vi "wav Crest Factor Analyzer.vi"() -> ()   [LabVIEW 2014]
doc: "This example demonstrates the effect of resampling a waveform in single-shot mode and the impact of the different resampling parameters. Single-shot mode is used when resampling a single block of the signal. Continuous mode is used when resampling separate but contiguous blocks of the signal."
uses:
  <vilib>/sound2/lvsound2.llb/Sound File Info (path).vi
  <vilib>/sound2/lvsound2.llb/Sound File Read Open.vi
  <vilib>/sound2/lvsound2.llb/Sound File Read (DBL).vi
  <vilib>/measure/maspectr.llb/FFT Spectrum (Mag-Phase) for N Chan.vi
  <vilib>/Utility/file.llb/Write To Spreadsheet File (string).vi
  <vilib>/Analysis/NI_AALPro.lvlib
  <vilib>/measure/NI_MAPro.lvlib
panel:
  in  "Auto Y":bool
  out "wav path":path
  out "FFT":cluster{"frequency":dbl[], "magnitude":dbl[]}[](graph)
  out "Result":string[][](array[string])
  in  "Tab Control":enum32{"General"}(tab)
  in  "Save":bool
  out "Progress bar":dbl(slide) scale=0.0..1.0
  in  "Analyze":bool
  out "Total no. of samples/ch":u32 format="%#_3p"
  out "Report path":path
  in  "Exit":bool
  in  "Smoothing":u16(ring)=3 items=["None"=0, "1/3 octave"=3, "1/6 octave"=6, "1/12 octave"=12, "1/24 octave"=24, "1/48 octave"=48]
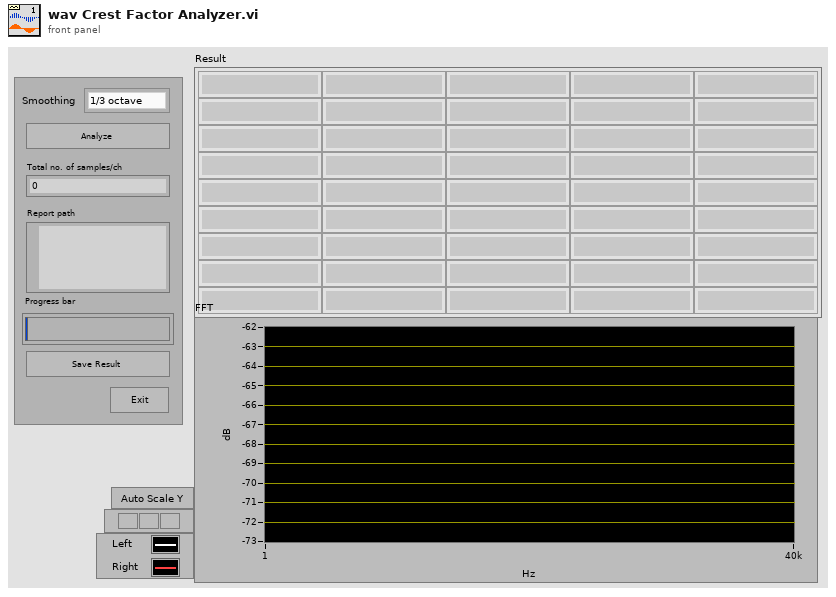
[diagram p1: front panel]
types:
  T1 = cluster{"averaging mode":enum16{"No averaging", "Vector averaging", "RMS averaging", "Peak hold"}, "weighting mode":enum16{"Linear", "Exponential"}, "number of averages":u32}
  T2 = cluster{"dB On (F)":bool, "unwrap phase (F)":bool, "convert to degree (F)":bool}
  T3 = typedef "Sound File Refnum.ctl" = refnum<file>
  T4 = typedef "imagedata.ctl" = cluster{"image type":i32, "image depth":i32, "image":u8[], "mask":u8[], "colors":u32[], "Rectangle":cluster{"left":i16, "top":i16, "right":i16, "bottom":i16}}
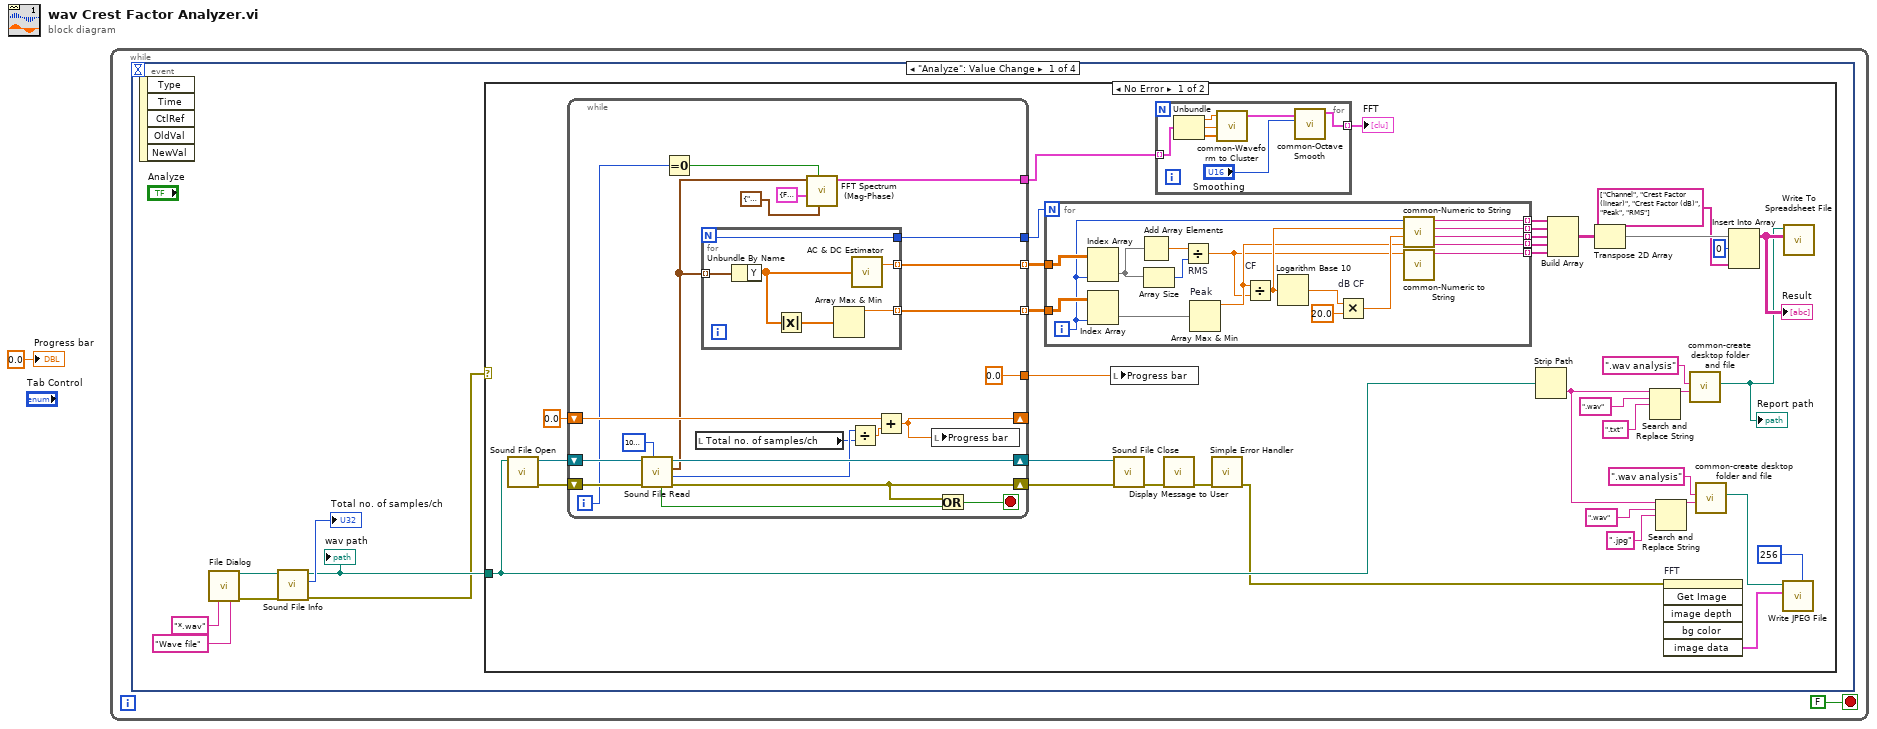
[diagram p0: block diagram]
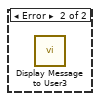
[diagram p2: hidden frame]
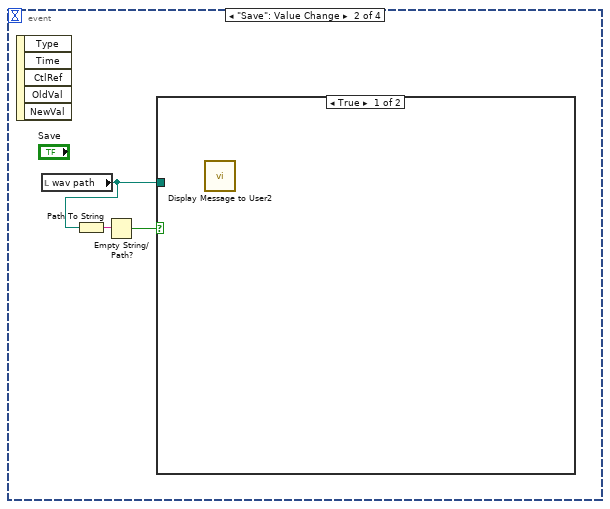
[diagram p3: hidden frame]
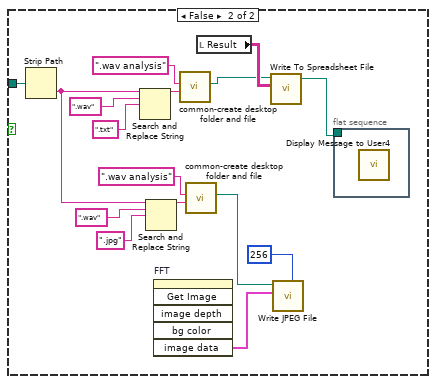
[diagram p4: hidden frame]
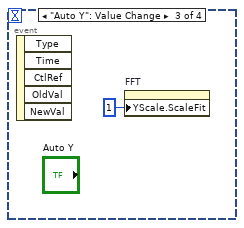
[diagram p5: hidden frame]
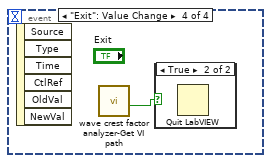
[diagram p6: hidden frame]
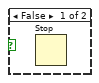
[diagram p7: hidden frame]
diagram:
  n1 = while {
    stop <- FALSE stop-if-true
    n2 = event shown="[0] \"Analyze\": Value Change" {
      selector: _ -> [_ _ _ _]
      dyn-events: _ -> [_ _ _ _]
      timeout: _ -> [_ _ _ _]
      event "Analyze": Value Change {
        n3 = event-data() -> ()  [unwired: 6 out]
        n4 = call "File Dialog"("pattern (all files)"="*.wav" ("pattern label"), "pattern label"="Wave file") -> ("selected path"=w7:path, "error out"=w4:errorcluster)  [unwired: 5 in, 7 out]
        n5 = call-poly <vilib>:"Sound File Info.vi"("error in (no error)"=w4, "path"=w7) -> ("error out"=w3:errorcluster, "total number of samples/ch"=→"Total no. of samples/ch":u32, "path out"=w5:path)  [unwired: 7 out]
        "wav path" <- w5
        n6 = case shown="No Error" w3 {
          tunnel: w5 -> [w22 _]
          frame No Error {
            n7 = call-poly <vilib>:"Sound File Open.vi"("path"=w22) -> ("error out"=w45:errorcluster, "sound file refnum"=w44:T3)  [unwired: 1 in, 8 out]
            n8 = while {
              shift-right: [w93] -> w47
              shift-left: w44 -> [w94]
              shift-right: [w75] -> w46
              shift-left: w45 -> [w92]
              shift-right: [w85] -> _
              shift-left: 0.0 ("Progress bar") -> [w90]
              tunnel: [0.0 ("Progress bar")] -> w42
              tunnel: [w84] -> w39 mode=indexing
              tunnel: [w83] -> w40 mode=indexing
              tunnel: [w82] -> w41
              tunnel: [w73] -> w10
              i -> [w80]
              stop <- w74 stop-if-true
              n9 = call-poly <vilib>:"Sound File Read.vi"("number of samples/ch (-1: all)"=1000000, "error in (no error)"=w92, "sound file refnum"=w94) -> ("error out"=w75:errorcluster, "offset"=w88:i32, "data"=w81:waveform(dbl)[], "sound file refnum out"=w93:T3, "end of file?"=w76:bool)  [unwired: 2 in, 2 out]
              n10 = Equal To 0?(x=w80) -> (x = 0?=w79:bool)
              n11 = local read "Total no. of samples/ch"() -> (w87:u32)
              n12 = for {
                N -> [w98]
                tunnel: w81 -> [w100] mode=indexing
                tunnel: [w99] -> w83 mode=indexing
                tunnel: [w97] -> w84 mode=indexing
                tunnel: [w98] -> w82
                n13 = Unbundle By Name(w100) -> ("Y"=w96:dbl[])
                n14 = Absolute Value(x=w96) -> (abs(x)=w95:dbl[])
                n15 = Array Max & Min(array=w95) -> (max value=w97:dbl)  [unwired: 3 out]
                n16 = call <vilib>:"AC & DC Estimator.vi"("Signal (V)"=w96) -> ("AC estimate (Vrms)"=w99:dbl)  [unwired: 1 out]
              }
              n17 = call-poly <vilib>:"FFT Spectrum (Mag-Phase).vi"("averaging parameters"=T1 {"averaging mode"=enum."No averaging", "weighting mode"=enum."Linear", "number of averages"=99999}, "restart averaging (F)"=w79, "view"=T2 {"dB On (F)"=FALSE, "unwrap phase (F)"=FALSE, "convert to degree (F)"=FALSE}, "time signals"=w81) -> ("magnitudes"=w73:cluster{"f0":dbl, "df":dbl, "magnitude":dbl[]}[])  [unwired: 3 in, 4 out]
              n18 = Divide(x=w88, y=w87) -> (x/y=w89:dbl)
              n19 = Add(x=w90, y=w89) -> (x+y=w85:dbl)
              n20 = local write "Progress bar"(w85) -> ()
              n21 = Or(x=w75, y=w76) -> (x .or. y?=w74:bool)
            }
            n22 = for {
              N: w41 -> [_]
              tunnel: w39 -> [w71]
              tunnel: w40 -> [w72]
              tunnel: [w59] -> w33 mode=indexing
              tunnel: [w58] -> w32 mode=indexing
              tunnel: [w57] -> w31 mode=indexing
              tunnel: [w56] -> w30 mode=indexing
              tunnel: [w55] -> w29 mode=indexing
              i -> [w64]
              n23 = Index Array(array=w72, index (col)=w64) -> (element=w69:dbl[])  [unwired: 1 in]
              n24 = Index Array(array=w71, index (col)=w64) -> (element=w70:dbl[])  [unwired: 1 in]
              n25 = Add Array Elements(numeric array=w69) -> (sum=w67:dbl)
              n26 = Array Size(array=w69) -> (size(s)=w68:i32)
              n27 = Divide "RMS"(x=w67, y=w68) -> (x/y=w60:dbl)
              n28 = Array Max & Min "Peak"(array=w70) -> (max value=w61:dbl)  [unwired: 3 out]
              n29 = Divide "CF"(x=w61, y=w60) -> (x/y=w62:dbl)
              n30 = Logarithm Base 10(1:w62) -> (0:w65:dbl)
              n31 = Multiply "dB CF"(x=w65, y=20.0) -> (x*y=w63:dbl)
              n32 = call "common-Numeric to String.vi"("Value 4"=w61, "Value 3"=w63, "Value 2"=w62, "Value 1"=w64) -> ("output string 4"=w56:string, "output string 3"=w57:string, "output string 2"=w58:string, "output string 1"=w59:string)  [unwired: 4 in]
              n33 = call "common-Numeric to String.vi"("Value 1"=w60) -> ("output string 1"=w55:string)  [unwired: 7 in, 3 out]
            }
            n34 = local write "Progress bar"(w42) -> ()
            n35 = call <vilib>:"Sound File Close.vi"("error in (no error)"=w46, "sound file refnum"=w47) -> ("error out"=w28:errorcluster)  [unwired: 9 out]
            n36 = for {
              tunnel: w10 -> [w54] mode=indexing
              tunnel: [w48] -> w20 mode=indexing
              n37 = Unbundle(w54) -> ("f0"=w51:dbl, "df"=w52:dbl, "magnitude"=w53:dbl[])
              n38 = call "common-Waveform to Cluster.vi"("Y"=w53, "dt, df"=w52, "t0, f0 (0)"=w51) -> ("Cluster out"=w50:cluster{"X":dbl[], "Y":dbl[]})  [unwired: 2 in]
              n39 = call "common-Octave Smooth.vi"("Smoothing (1/24)"="Smoothing", "Input data"=w50) -> ("Output Data"=w48:cluster{"frequency":dbl[], "magnitude":dbl[]})  [unwired: 9 in]
            }
            "FFT" <- w20
            n40 = call "Display Message to User"("error in (no error)"=w28) -> ("error out"=w27:errorcluster)  [unwired: 9 in, 1 out]
            n41 = call <vilib>:"Simple Error Handler.vi"("error in (no error)"=w27) -> ("error out"=w18:errorcluster)  [unwired: 1 in, 7 out]
            n42 = Strip Path(path=w22) -> (name=w13:string)  [unwired: 1 out]
            n43 = Build Array(w33, w32, w31, w30, w29) -> (w38:string[][])
            n44 = Transpose 2D Array(2D array=w38) -> (transposed array=w37:string[][])
            n45 = Search and Replace String(input string=w13, search string=".wav", replace string=".txt" ("replace string (\"\")")) -> (result string=w23:string)  [unwired: 5 in, 3 out]
            n46 = Search and Replace String(input string=w13, search string=".wav", replace string=".jpg" ("replace string (\"\")")) -> (result string=w17:string)  [unwired: 5 in, 3 out]
            n47 = invoke on="FFT" class="XYGraph (strict)" method="Get Image"(error in=w18) -> ("image data"=w19:T4)  [unwired: 5 in, 5 out]
            n48 = call "common-create desktop folder and file.vi"("File Name"=w23, "Folder Name"=".wav analysis") -> ("file path"=w21:path)  [unwired: 9 in]
            "Report path" <- w21
            n49 = call "common-create desktop folder and file.vi"("File Name"=w17, "Folder Name"=".wav analysis") -> ("file path"=w12:path)  [unwired: 9 in]
            n50 = Insert Into Array(array=w37, index (row)=0, new element=string[] ["Channel", "Crest Factor (linear)", "Crest Factor (dB)", "Peak", "RMS"] ("Name")) -> (w34:string[][])  [unwired: 1 in]
            "Result" <- w34
            n51 = call <vilib>:"Write JPEG File.vi"("quality (80)"=256, "image data"=w19, "path to JPEG file"=w12) -> ()  [unwired: 7 in, 2 out]
            n52 = call-poly <vilib>:"Write To Spreadsheet File.vi"("2D data"=w34, "file path (dialog if empty)"=w21) -> ()  [unwired: 6 in, 1 out]
          }
          frame Error {
            n53 = call "Display Message to User3"() -> ()  [unwired: 10 in, 2 out]
          }
        }
      }
      event "Save": Value Change {
        n54 = event-data() -> ()  [unwired: 6 out]
        n55 = local read "wav path"() -> (w102:path)
        n56 = Path To String(path=w102) -> (string=w103:string)
        n57 = Empty String/Path?(string/path=w103) -> (empty?=w101:bool)
        n58 = case shown="True" w101 {
          tunnel: w102 -> [_ w106]
          frame True {
            n59 = call "Display Message to User2"() -> ()  [unwired: 10 in, 2 out]
          }
          frame False {
            n60 = Strip Path(path=w106) -> (name=w110:string)  [unwired: 1 out]
            n61 = Search and Replace String(input string=w110, search string=".wav", replace string=".txt" ("replace string (\"\")")) -> (result string=w116:string)  [unwired: 5 in, 3 out]
            n62 = Search and Replace String(input string=w110, search string=".wav", replace string=".jpg" ("replace string (\"\")")) -> (result string=w114:string)  [unwired: 5 in, 3 out]
            n63 = invoke on="FFT" class="XYGraph (strict)" method="Get Image"() -> ("image data"=w115:T4)  [unwired: 6 in, 5 out]
            n64 = call "common-create desktop folder and file.vi"("File Name"=w116, "Folder Name"=".wav analysis") -> ("file path"=w107:path)  [unwired: 9 in]
            n65 = call "common-create desktop folder and file.vi"("File Name"=w114, "Folder Name"=".wav analysis") -> ("file path"=w109:path)  [unwired: 9 in]
            n66 = local read "Result"() -> (w108:string[][])
            n67 = call-poly <vilib>:"Write To Spreadsheet File.vi"("2D data"=w108, "file path (dialog if empty)"=w107) -> ("new file path (Not A Path if cancelled)"=w105:path)  [unwired: 6 in]
            n68 = call <vilib>:"Write JPEG File.vi"("quality (80)"=256, "image data"=w115, "path to JPEG file"=w109) -> ()  [unwired: 7 in, 2 out]
            n69 = flat-sequence {
              tunnel: w105 -> [_]
              frame #0 {
                n70 = call "Display Message to User4"() -> ()  [unwired: 10 in, 2 out]
              }
            }
          }
        }
      }
      event "Auto Y": Value Change {
        n71 = event-data() -> ()  [unwired: 6 out]
        n72 = property on="FFT" class="XYGraph (strict)"("YScale.ScaleFit"=u8 1 ("Y Scale.Scale Fit")) -> ()  [unwired: 2 in, 2 out]
      }
      event "Exit": Value Change {
        n73 = event-data() -> ()  [unwired: 7 out]
        n74 = call "wave crest factor analyzer-Get VI path.vi"() -> ("Is exe?"=w121:bool)  [unwired: 9 in, 2 out]
        n75 = case shown="True" w121 {
          frame False {
            n76 = Stop() -> ()  [unwired: 1 in]
          }
          frame True {
            n77 = Quit LabVIEW() -> ()  [unwired: 1 in]
          }
        }
      }
    }
  }
  "Progress bar" <- 0.0 ("Progress bar")
